vi "Test_Settings_Sequence_Params.vi"() -> ()   [LabVIEW 2015]
uses:
  controls/SEQUENCE_UI_Inputs.ctl
panel:
  out "SEQUENCE 2":T1
  out "sortie d'erreur":errorcluster
  in  "stop":bool
  in  "Bouton CANCEL":bool
  in  "Bouton OK":bool
  in  "SEQUENCE":T1
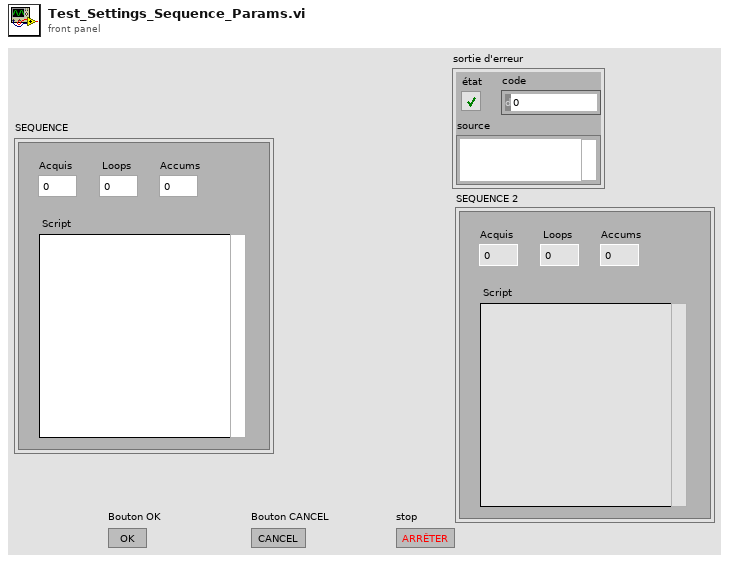
[diagram p1: front panel]
types:
  T1 = typedef "SEQUENCE_UI_Inputs.ctl" = cluster{"Loops":i16, "Accums":i16, "Script":string, " Acquis":i16}
  T2 = enum8{"Enabled", "Disabled", "Disabled and Grayed Out"}
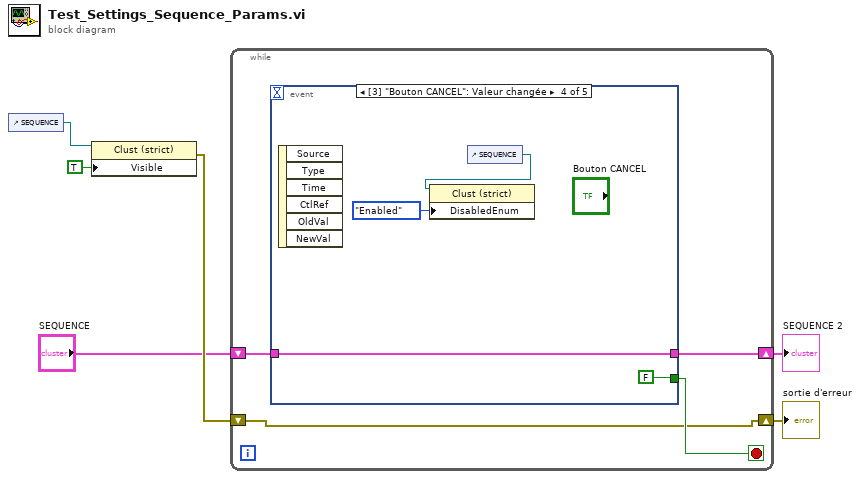
[diagram p0: block diagram]
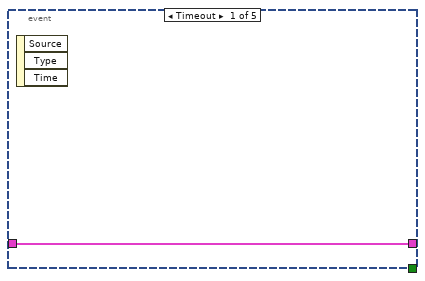
[diagram p2: hidden frame]
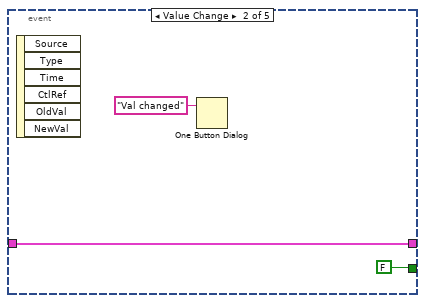
[diagram p3: hidden frame]
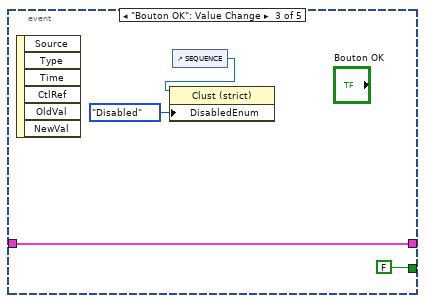
[diagram p4: hidden frame]
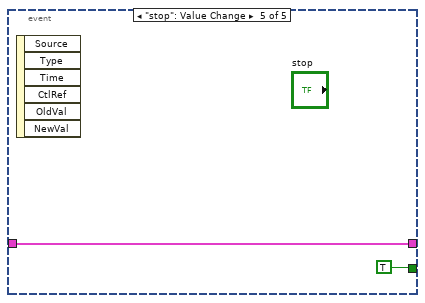
[diagram p5: hidden frame]
diagram:
  n1 = control-ref of="SEQUENCE"() -> (w5:refnum<vi>)
  n2 = property class="Clust (strict)"(reference=w5, "Visible"=TRUE) -> (error out=w4:errorcluster)  [unwired: 1 in, 1 out]
  n3 = while {
    shift-right: [w9] -> w3
    shift-left: w4 -> [w9]
    shift-right: [w7] -> w1
    shift-left: "SEQUENCE" -> [w8]
    stop <- w10 stop-if-true
    n4 = event shown="[3] \"Bouton CANCEL\": Valeur changée" {
      selector: _ -> [_ _ _ _ _]
      dyn-events: _ -> [_ _ _ _ _]
      timeout: _ -> [_ _ _ _ _]
      tunnel: [_ FALSE FALSE FALSE TRUE] -> w10
      tunnel: w8 -> [w11 w12 w16 w20 w23]
      tunnel: [w11 w12 w16 w20 w23] -> w7
      event Timeout {
        n5 = event-data() -> ()  [unwired: 1 in, 3 out]
      }
      event Value Change {
        n6 = event-data() -> ()  [unwired: 1 in, 6 out]
        n7 = One Button Dialog(message="Val changed") -> ()  [unwired: 1 in, 1 out]
      }
      event "Bouton OK": Value Change {
        n8 = event-data() -> ()  [unwired: 1 in, 6 out]
        n9 = control-ref of="SEQUENCE"() -> (w17:refnum<vi>)
        n10 = property class="Clust (strict)"(reference=w17, "DisabledEnum"=T2."Disabled" ("Désactivé")) -> ()  [unwired: 1 in, 2 out]
      }
      event "Bouton CANCEL": Value Change {
        n11 = event-data() -> ()  [unwired: 1 in, 6 out]
        n12 = control-ref of="SEQUENCE"() -> (w21:refnum<vi>)
        n13 = property class="Clust (strict)"(reference=w21, "DisabledEnum"=T2."Enabled" ("Désactivé")) -> ()  [unwired: 1 in, 2 out]
      }
      event "stop": Value Change {
        n14 = event-data() -> ()  [unwired: 1 in, 6 out]
      }
    }
  }
  "sortie d'erreur" <- w3
  "SEQUENCE 2" <- w1
